vi "labview tania 3.vi"() -> ()   [LabVIEW 2011]
panel:
  out "Menor":dbl
  out "Mayor":dbl
  out "Promedio":dbl
  out "Temperatura":dbl(slide) scale=0.0..100.0
  # "Generar 10 temperaturas y al final presentar la temperatura mayor, menor y la temperatura promedio."
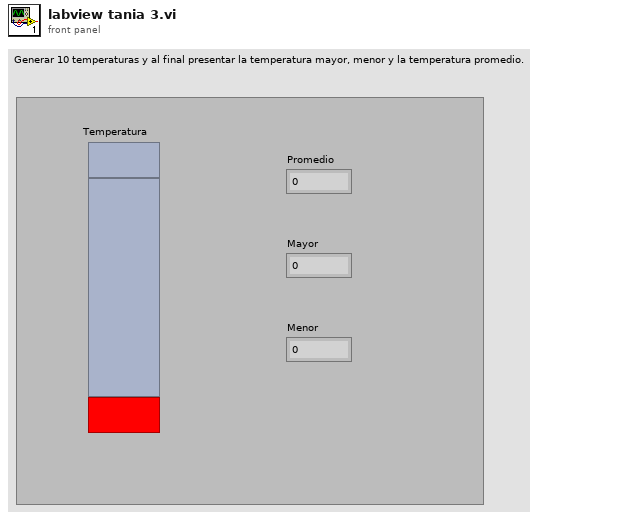
[diagram p1: front panel]
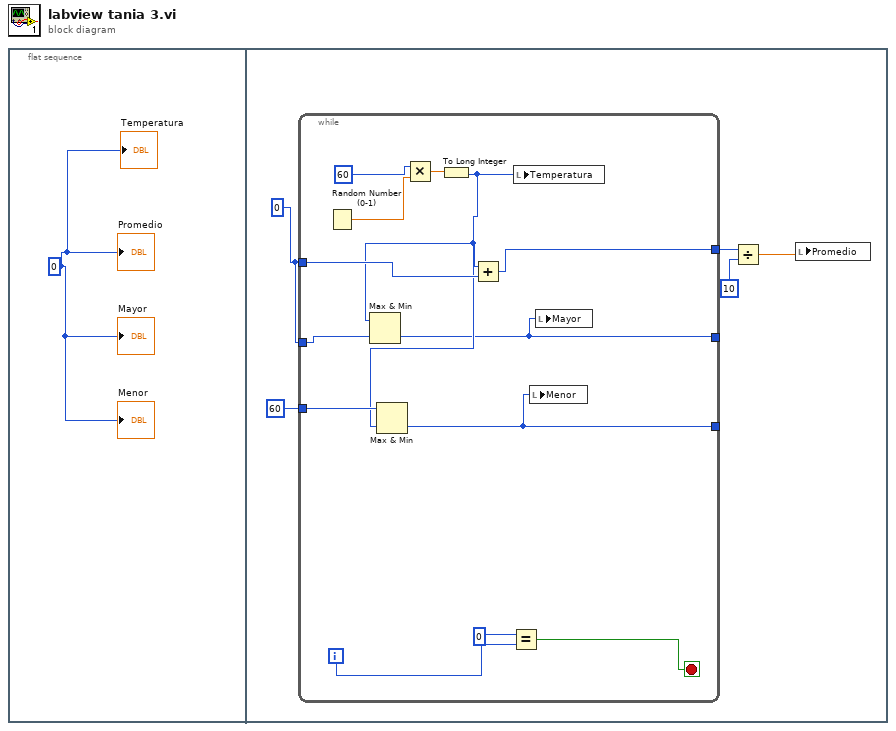
[diagram p0: block diagram]
diagram:
  n1 = flat-sequence {
    frame #0 {
      w1 = 0
      "Temperatura" <- w1
      "Promedio" <- w1
      "Mayor" <- w1
      "Menor" <- w1
    }
    frame #1 {
      w3 = 0
      n2 = while {
        tunnel: w3 -> [w13]
        tunnel: [w12] -> w6
        tunnel: w3 -> [w11]
        tunnel: 60 -> [w10]
        tunnel: [w7] -> _
        tunnel: [w8] -> _
        i -> [w19]
        stop <- w17 stop-if-true
        n3 = Random Number (0-1)() -> (number: 0 to 1=w15:dbl)
        n4 = Multiply(x=60, y=w15) -> (x*y=w14:dbl)
        n5 = To Long Integer(number=w14) -> (32bit integer=w9:i32)
        n6 = Max & Min(x=w9, y=w11) -> (min(x,y)=w8:i32)  [unwired: 1 out]
        n7 = Max & Min(x=w10, y=w9) -> (min(x,y)=w7:i32)  [unwired: 1 out]
        n8 = Add(x=w9, y=w13) -> (x+y=w12:i32)
        n9 = Equal?(x=w19, y=0) -> (x = y?=w17:bool)
        n10 = local write "Temperatura"(w9) -> ()
        n11 = local write "Menor"(w7) -> ()
        n12 = local write "Mayor"(w8) -> ()
      }
      n13 = Divide(x=w6, y=10) -> (x/y=w4:dbl)
      n14 = local write "Promedio"(w4) -> ()
    }
  }
